vi "Export Plugin Configuration.vi"(8 "error in":errorcluster, 10 "Path":path, 11 "Device Item Ref in":T1 format="%.0x") -> (0 "error out":errorcluster, 3 "Device Item Ref out":T1 format="%.0x")   [LabVIEW 2026, in "Template System Explorer.lvlib"]
uses:
  Template System Explorer.lvlib
  NationalInstruments.VeriStand.SystemDefinitionAPI
  <vilib>/NI VeriStand/Custom Device API/Custom Device Item Ref.ctl
  <vilib>/NI VeriStand/Custom Device API/Custom Device API.lvlib
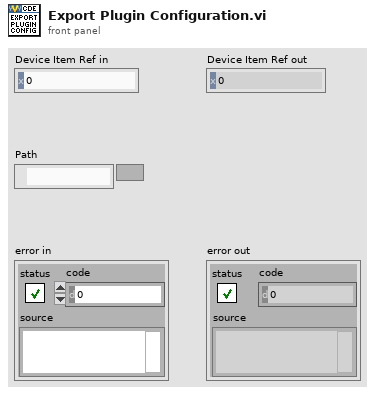
[diagram p1: front panel]
types:
  T1 = typedef "Custom Device API.lvlib/Custom Device Item Ref.ctl" = u64
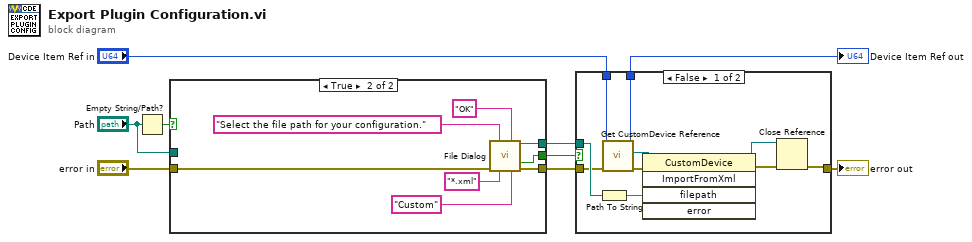
[diagram p0: block diagram]
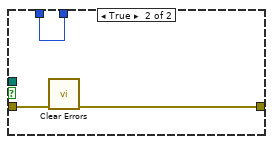
[diagram p2: hidden frame]
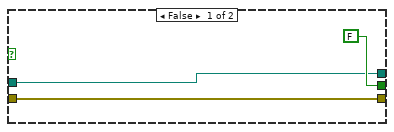
[diagram p3: hidden frame]
diagram:
  n1 = Empty String/Path?(string/path="Path") -> (empty?=w6:bool)
  n2 = case shown="True" w6 {
    tunnel: [FALSE ("cancelled") w15] -> w4
    tunnel: [w12 w20] -> w8
    tunnel: [w10 w14] -> w3
    tunnel: "error in" -> [w12 w19]
    tunnel: "Path" -> [w10 _]
    frame False {
    }
    frame True {
      n3 = call "File Dialog"("prompt"="Select the file path for your configuration.", "button label"="OK", "error in"=w19, "pattern (all files)"="*.xml", "pattern label"="Custom") -> ("selected path"=w14:path, "cancelled"=w15:bool, "error out"=w20:errorcluster)  [unwired: 7 in, 1 out]
    }
  }
  n4 = case shown="False" w4 {
    tunnel: [w23 w32] -> w7
    tunnel: w8 -> [w26 w33]
    tunnel: "Device Item Ref in" -> [w27 w31]
    tunnel: w3 -> [w30 _]
    tunnel: [w22 w31] -> w1
    frame False {
      n5 = Path To String(path=w30) -> (string=w21:string)
      n6 = call "Get CustomDevice Reference.vi"("error in"=w26, "Node Ptr"=w27) -> ("error out"=w25:errorcluster, "Custom Device"=w28:refnum<k24>, "Node Ptr"=w22:T1)  [unwired: 7 in]
      n7 = invoke class="CustomDevice" method="ImportFromXml"(reference=w28, error in=w25, "filepath"=w21) -> (reference out=w29:refnum<k24>, error out=w24:errorcluster)  [unwired: 2 in, 3 out]
      n8 = Close Reference(reference=w29, error in (no error)=w24) -> (error out=w23:errorcluster)
    }
    frame True {
      n9 = call <vilib>:"Clear Errors.vi"("error in (no error)"=w33) -> ("error out"=w32:errorcluster)  [unwired: 5 in, 1 out]
    }
  }
  "error out" <- w7
  "Device Item Ref out" <- w1
